vi "CS POLARIS BME DG Client.destructor.vi"(0 "i ref in":refnum<vi>, 5 "error in (no error)":errorcluster) -> (19 "error out":errorcluster)   [LabVIEW 2009, in "CS POLARIS BME DG Client.lvlib"]
doc: "This is the destructor of a class.\n\nLicense Agreement for this software:\n\nCopyright (C)\nGesellschaft für Schwerionenforschung, GSI\nPlanckstr. 1\n64291 Darmstadt\nGermany\n\nContact: D.Beck@gsi.de \n\nThis program is free software; you can redistribute it and/or modify it under the terms of the \nGNU General Public License as published by the Free Software Foundation; either version 2 of \nthe license, or (at your option) any later version.\n\nThis program is distributed in the hope that it will be useful, but WITHOUT ANY WARRANTY; \nwithout even the implied warranty of MERCHANTABILITY or FITNESS FOR A PARTICULAR PURPOSE. See the GNU General License for more details (http://www.gnu.org).\n\nGesellschaft für Schwerionenforschung, GSI\nPlanckstr. 1, 64291 Darmstadt, Germany\nFor all questions and ideas contact: M.Richter@gsi.de, H.Brand@gsi.de or D.Beck@gsi.de.\nLast update: 16-JUN-2004"
uses:
  CS POLARIS BME DG Client.lvlib
  CSCore/BaseProcess/BaseProcess.lvlib
  CSCore/BaseGUI/BaseGUI.lvlib
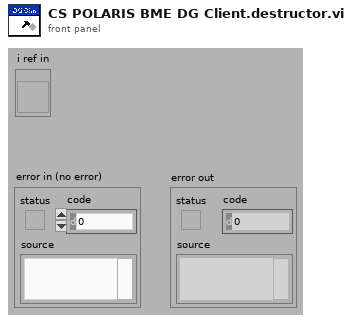
[diagram p1: front panel]
types:
  T1 = typedef "CS POLARIS BME DG Client.lvlib/CS POLARIS BME DG Client.i attribute.ctl" = cluster{"Delay Formula Ref":refnum<vi>, "Active Ref":refnum<vi>, "OutputModulo Ref":refnum<vi>, "Rep Rate Ref":refnum<vi>, "Next Shot Ref":refnum<vi>, "Error Ref":refnum<vi>, "Switch Ref":refnum<vi>, "New Delay Formula Ref":refnum<vi>, "New OutputModulo Ref ":refnum<vi>, "Channel":string, "CS DG Obj":string, "Stop Ref":refnum<vi>, "Max delay change":dbl, "Enabled fields":u8, "LockInfo Ref":refnum<vi>}
  T2 = enum16{"SetAttribute", "GetAttribute", "CreateAttribute", "DestroyAttribute", "DestroyAllAtributes"}
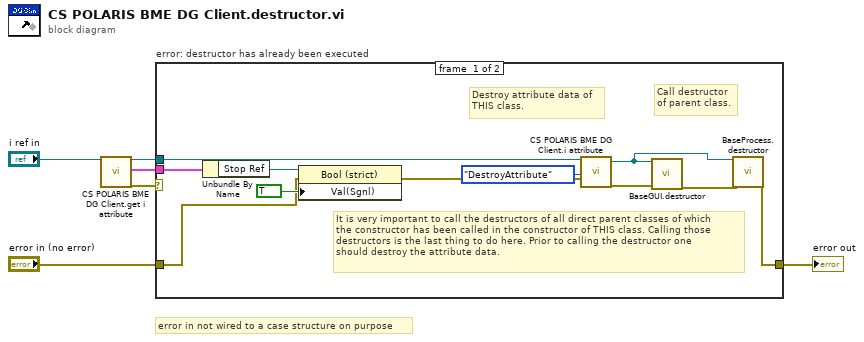
[diagram p0: block diagram]
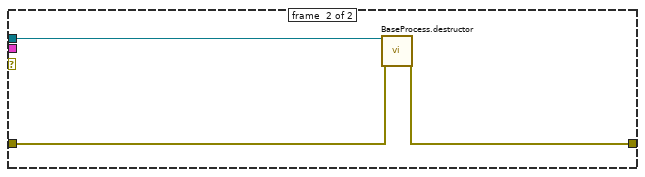
[diagram p2: hidden frame]
diagram:
  # "error in not wired to a case structure on purpose"
  n1 = call "CS POLARIS BME DG Client.get i attribute.vi"("i ref in"="i ref in") -> ("i ref out"=w2:refnum<vi>, "i attribute"=w1:T1, "error out"=w3:errorcluster)  [unwired: 16 in]
  n2 = case "error: destructor has already been executed" shown="No Error" w3 {
    tunnel: [w16 w18] -> w6
    tunnel: "error in (no error)" -> [w8 w19]
    tunnel: w2 -> [w15 w20]
    tunnel: w1 -> [w11 _]
    frame #0 {
      # "It is very important to call the destructors of all direct parent classes of which\nthe constructor has been called in the constructor of THIS class. Calling those\ndestructors is the last thing to do here. Prior to calling the destructor one \nshould destroy the attribute data."
      # "Destroy attribute data of \nTHIS class."
      # "Call destructor\nof parent class."
      n3 = Unbundle By Name(w11) -> ("Stop Ref"=w10:refnum<vi>)
      n4 = property class="Bool (strict)"(reference=w10, error in=w8, "Val(Sgnl)"=TRUE ("Value (Signaling)")) -> (error out=w7:errorcluster)  [unwired: 1 out]
      n5 = call "CS POLARIS BME DG Client.i attribute.vi"("VI Refnum"=w15, "Action"=T2."DestroyAttribute", "error in (no error)"=w7) -> ("VI Refnum out"=w12:refnum<vi>, "error out"=w14:errorcluster)  [unwired: 14 in, 1 out]
      n6 = call "BaseGUI.destructor.vi"("i ref in"=w12, "error in (no error)"=w14) -> ("error out"=w13:errorcluster)  [unwired: 17 in]
      n7 = call "BaseProcess.destructor.vi"("i ref in"=w12, "error in (no error)"=w13) -> ("error out"=w16:errorcluster)  [unwired: 17 in]
    }
    frame #1 {
      n8 = call "BaseProcess.destructor.vi"("i ref in"=w20, "error in (no error)"=w19) -> ("error out"=w18:errorcluster)  [unwired: 17 in]
    }
  }
  "error out" <- w6
